vi "UTILITY Delete Empty String Cells.vi"(11 "Array with Empty Cells":string[](array[string])) -> (3 "Array w/o Empty Cells":string[](array[string]))   [LabVIEW 2018]
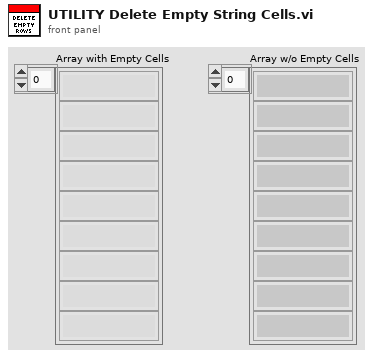
[diagram p1: front panel]
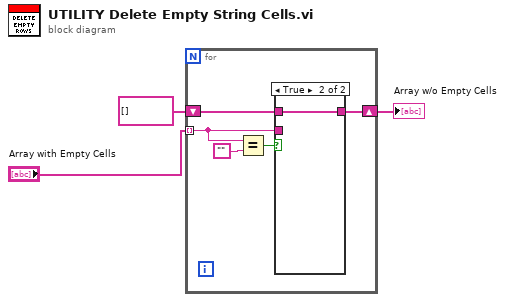
[diagram p0: block diagram]
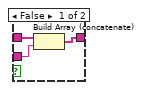
[diagram p2: hidden frame]
diagram:
  n1 = for {
    tunnel: "Array with Empty Cells" -> [w5] mode=indexing
    shift-right: [w4] -> w3
    shift-left: string[] [] -> [w6]
    n2 = Equal?(x=w5, y="") -> (x = y?=w7:bool)
    n3 = case shown="True" w7 {
      tunnel: w6 -> [w11 w12]
      tunnel: w5 -> [w10 _]
      tunnel: [w9 w12] -> w4
      frame False {
        n4 = Build Array (concatenate)(w11, w10) -> (w9:string[])
      }
      frame True {
      }
    }
  }
  "Array w/o Empty Cells" <- w3
